vi "sensor_messung.vi"(8 "error in (no error)":errorcluster, 10 "Sensorkoord [P1 P2]":dbl[][](array[numeric]), 11 "Gerade in":refnum<class "Gerade.lvclass">) -> (0 "error out":errorcluster, 1 "Sensor auf Linie":bool, 2 "Schnittpunkt":dbl[](array[numeric]), 3 "Gerade out":refnum<class "Gerade.lvclass">)   [LabVIEW 2019, in "Gerade.lvclass"]
uses:
  Gerade.lvclass
  Gerade.lvclass/Gerade.ctl
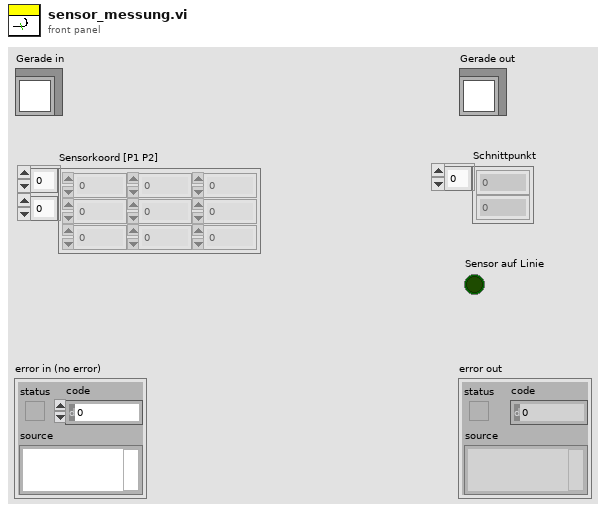
[diagram p1: front panel]
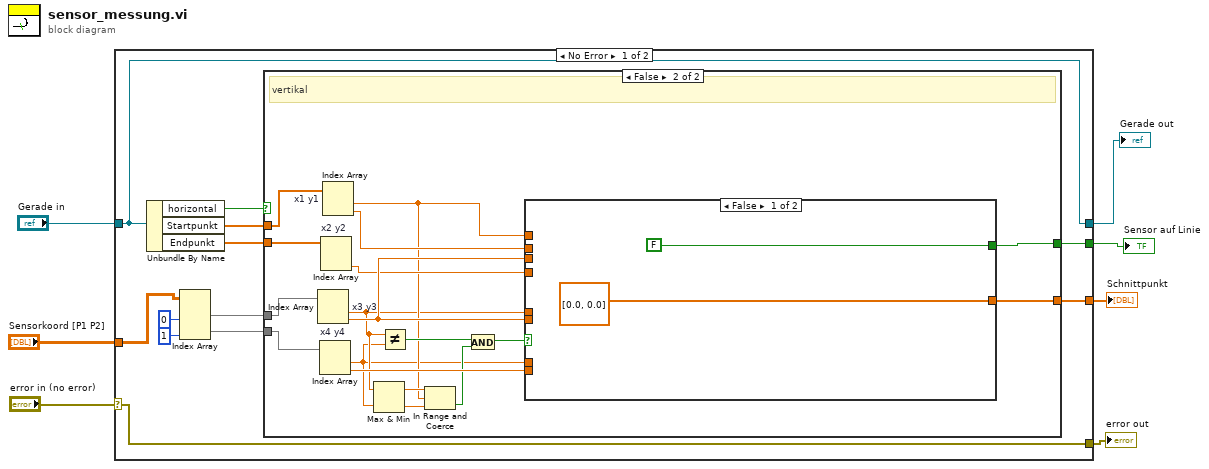
[diagram p0: block diagram]
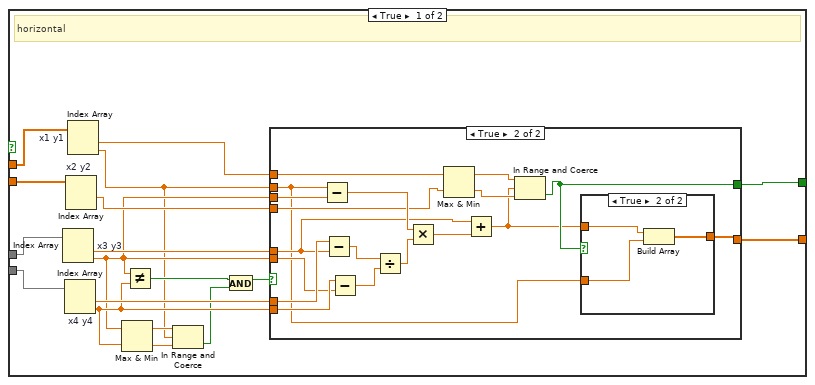
[diagram p2: hidden frame]
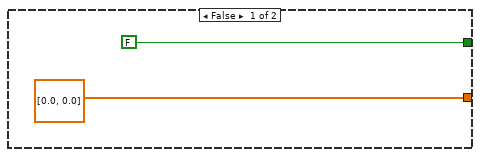
[diagram p3: hidden frame]
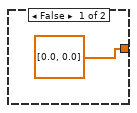
[diagram p4: hidden frame]
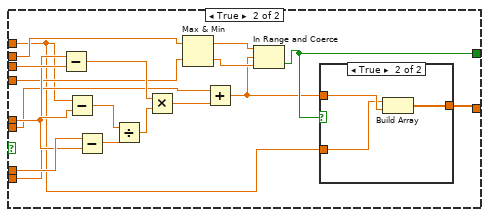
[diagram p5: hidden frame]
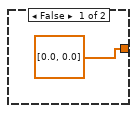
[diagram p6: hidden frame]
diagram:
  n1 = case shown="No Error" "error in (no error)" {
    selector: "error in (no error)" -> [w9 w105]
    tunnel: "Gerade in" -> [w8 w104]
    tunnel: "Sensorkoord [P1 P2]" -> [w18 _]
    tunnel: [w13 _] -> w4
    tunnel: [w12 _] -> w3
    tunnel: [w9 w105] -> w2
    tunnel: [w8 w104] -> w1
    frame No Error {
      n2 = Unbundle By Name(w8) -> ("horizontal"=w19:bool, "Startpunkt"=w11:dbl[], "Endpunkt"=w10:dbl[])
      n3 = Index Array(array=w18, index (col) #1=0 ("disabled index (col)"), index (col) #2=1 ("index (col)")) -> (element #1=w15:dbl[], element #2=w14:dbl[])  [unwired: 2 in]
      n4 = case shown="False" w19 {
        tunnel: w15 -> [w37 w79]
        tunnel: w14 -> [w36 w78]
        tunnel: [w32 w75] -> w13
        tunnel: [w31 w74] -> w12
        tunnel: w11 -> [w30 w73]
        tunnel: w10 -> [w29 w72]
        frame True {
          # "horizontal"
          n5 = Index Array "x3 y3"(array=w37) -> (element #1=w34:dbl, element #2=w23:dbl)  [unwired: 2 in]
          n6 = Index Array "x4 y4"(array=w36) -> (element #1=w35:dbl, element #2=w24:dbl)  [unwired: 2 in]
          n7 = Index Array "x2 y2"(array=w29) -> (element #1=w27:dbl)  [unwired: 2 in, 1 out]
          n8 = Index Array "x1 y1"(array=w30) -> (element #1=w28:dbl, element #2=w22:dbl)  [unwired: 2 in]
          n9 = Max & Min(x=w23, y=w24) -> (max(x,y)=w26:dbl, min(x,y)=w25:dbl)
          n10 = Not Equal?(x=w23, y=w24) -> (x != y?=w33:bool)
          n11 = In Range and Coerce(upper limit=w26, x=w22, lower limit=w25) -> (In Range?=w20:bool)  [unwired: 1 out]
          n12 = And(x=w33, y=w20) -> (x .and. y?=w21:bool)
          n13 = case shown="True" w21 {
            tunnel: w35 -> [_ w57]
            tunnel: w34 -> [_ w49]
            tunnel: w24 -> [_ w54]
            tunnel: w23 -> [_ w53]
            tunnel: [FALSE w43] -> w32
            tunnel: [dbl[] [0.0, 0.0] w40] -> w31
            tunnel: w22 -> [_ w41]
            tunnel: w23 -> [_ w52]
            tunnel: w28 -> [_ w47]
            tunnel: w27 -> [_ w46]
            frame False {
            }
            frame True {
              n14 = Subtract(x=w41, y=w52) -> (x-y=w50:dbl)
              n15 = Subtract(x=w57, y=w49) -> (x-y=w56:dbl)
              n16 = Subtract(x=w54, y=w53) -> (x-y=w55:dbl)
              n17 = Divide(x=w56, y=w55) -> (x/y=w51:dbl)
              n18 = Multiply(x=w50, y=w51) -> (x*y=w48:dbl)
              n19 = Max & Min(x=w47, y=w46) -> (max(x,y)=w44:dbl, min(x,y)=w45:dbl)
              n20 = Add(x=w49, y=w48) -> (x+y=w42:dbl)
              n21 = In Range and Coerce(upper limit=w44, x=w42, lower limit=w45) -> (In Range?=w43:bool)  [unwired: 1 out]
              n22 = case shown="True" w43 {
                tunnel: w42 -> [_ w61]
                tunnel: w41 -> [_ w60]
                tunnel: [dbl[] [0.0, 0.0] w59] -> w40
                frame False {
                }
                frame True {
                  n23 = Build Array(w61, w60) -> (w59:dbl[])
                }
              }
            }
          }
        }
        frame False {
          # "vertikal"
          n24 = Index Array "x3 y3"(array=w79) -> (element #1=w63:dbl, element #2=w70:dbl)  [unwired: 2 in]
          n25 = Index Array "x4 y4"(array=w78) -> (element #1=w62:dbl, element #2=w77:dbl)  [unwired: 2 in]
          n26 = Index Array "x2 y2"(array=w72) -> (element #2=w69:dbl)  [unwired: 2 in, 1 out]
          n27 = Index Array "x1 y1"(array=w73) -> (element #1=w64:dbl, element #2=w71:dbl)  [unwired: 2 in]
          n28 = Max & Min(x=w63, y=w62) -> (max(x,y)=w68:dbl, min(x,y)=w67:dbl)
          n29 = Not Equal?(x=w63, y=w62) -> (x != y?=w76:bool)
          n30 = In Range and Coerce(upper limit=w68, x=w64, lower limit=w67) -> (In Range?=w65:bool)  [unwired: 1 out]
          n31 = And(x=w76, y=w65) -> (x .and. y?=w66:bool)
          n32 = case shown="False" w66 {
            tunnel: w62 -> [_ w99]
            tunnel: w63 -> [_ w87]
            tunnel: w77 -> [_ w86]
            tunnel: w70 -> [_ w85]
            tunnel: [FALSE w90] -> w75
            tunnel: [dbl[] [0.0, 0.0] w88] -> w74
            tunnel: w71 -> [_ w84]
            tunnel: w70 -> [_ w96]
            tunnel: w64 -> [_ w82]
            tunnel: w69 -> [_ w83]
            frame False {
            }
            frame True {
              n33 = Subtract(x=w86, y=w96) -> (x-y=w94:dbl)
              n34 = Subtract(x=w82, y=w87) -> (x-y=w97:dbl)
              n35 = Subtract(x=w99, y=w87) -> (x-y=w98:dbl)
              n36 = Divide(x=w97, y=w98) -> (x/y=w95:dbl)
              n37 = Multiply(x=w94, y=w95) -> (x*y=w93:dbl)
              n38 = Max & Min(x=w84, y=w83) -> (max(x,y)=w91:dbl, min(x,y)=w92:dbl)
              n39 = Add(x=w85, y=w93) -> (x+y=w89:dbl)
              n40 = In Range and Coerce(upper limit=w91, x=w89, lower limit=w92) -> (In Range?=w90:bool)  [unwired: 1 out]
              n41 = case shown="True" w90 {
                tunnel: w89 -> [_ w103]
                tunnel: w82 -> [_ w102]
                tunnel: [dbl[] [0.0, 0.0] w101] -> w88
                frame False {
                }
                frame True {
                  n42 = Build Array(w102, w103) -> (w101:dbl[])
                }
              }
            }
          }
        }
      }
    }
    frame Error {
    }
  }
  "error out" <- w2
  "Gerade out" <- w1
  "Schnittpunkt" <- w3
  "Sensor auf Linie" <- w4
